vi "Obtain Queue.vi"(8 "error in (no error)":errorcluster, 9 "Region":T1, 10 "Name":string, 11 "AWS Credentials":T2) -> (0 "error out":errorcluster, 3 "SQS":refnum<class "NI_AWS_SQS.lvclass">)   [LabVIEW 2015, in "NI_AWS_SQS.lvclass"]
uses:
  NI_AWS_SQS.lvclass
  Core/AWS Credentials.ctl
  Core/Region.ctl
  NI_AWS_SQS.lvclass/NI_AWS_SQS.ctl
  Read Name.vi
  <vilib>/Utility/error.llb/Error Cluster From Error Code.vi
  <vilib>/ErrorRing/Error Ring.xnode
  Core/NI_AWS_Core.lvclass
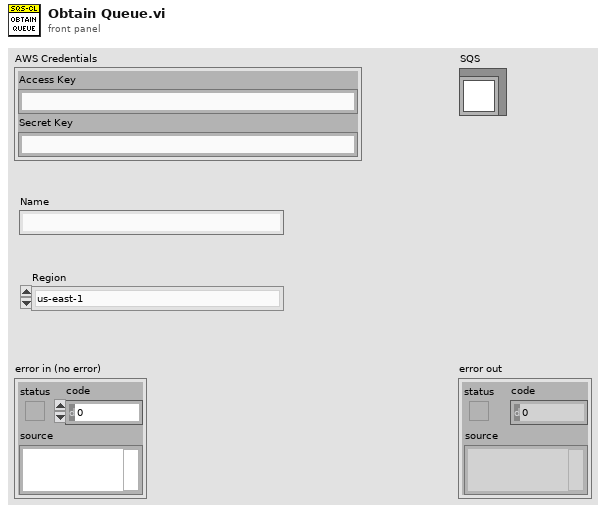
[diagram p1: front panel]
types:
  T1 = typedef "NI_AWS_Core.lvclass/Region.ctl" = enum16{"us-east-1", "us-east-2", "us-west-1", "us-west-2", "ap-northeast-1", "ap-northeast-2", "ap-southeast-1", "ap-southeast-2", "ca-central-1", "eu-central-1", "eu-west-1", "eu-west-2", "sa-east-1"}
  T2 = typedef "NI_AWS_Core.lvclass/AWS Credentials.ctl" = cluster{"Access Key":string, "Secret Key":string}
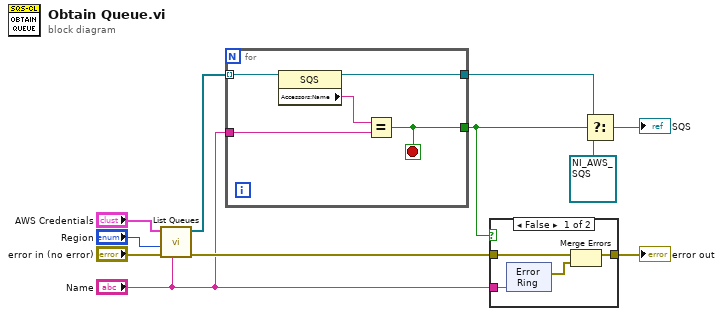
[diagram p0: block diagram]
diagram:
  n1 = call "List Queues.vi"("Name Prefix"="Name", "error in (no error)"="error in (no error)", "Region"="Region", "AWS Credentials"="AWS Credentials") -> ("error out"=w3:errorcluster, "SQS Queues"=w8:refnum<class "NI_AWS_SQS.lvclass">[])  [unwired: 6 in]
  n2 = for {
    tunnel: w8 -> [w16] mode=indexing
    tunnel: "Name" -> [w14]
    tunnel: [w13] -> w4
    tunnel: [w12] -> w7
    stop <- w13 stop-if-true
    n3 = property class="SQS"(reference=w16) -> (reference out=w12:refnum<class "NI_AWS_SQS.lvclass">, "Accessors:Name"=w15:string)  [unwired: 1 in, 1 out]
    n4 = Equal?(x=w15, y=w14) -> (x = y?=w13:bool)
  }
  n5 = case shown="False" w4 {
    tunnel: w3 -> [w20 w28]
    tunnel: [w19 w28] -> w2
    tunnel: "Name" -> [w17 _]
    frame False {
      n6 = xnode "Error Ring"("parameter 0"=w17) -> ("error out"=w18:errorcluster)
      n7 = Merge Errors(w20, w18) -> (w19:errorcluster)
    }
    frame True {
    }
  }
  "error out" <- w2
  n8 = Select(t=w7, s=w4, f=refnum<class "NI_AWS_SQS.lvclass"> refnum ("NI_SQS.lvlib:SQS")) -> (s? t:f=→"SQS":refnum<class "NI_AWS_SQS.lvclass">)
